vi "Register Listener.vi"(8 "error in (no error)":errorcluster, 10 "Actor's Enqueuer":refnum<class "Message Enqueuer.lvclass">, 11 "Trace Controller in":refnum<class "Trace Controller.lvclass">) -> (0 "error out":errorcluster, 3 "Trace Controller out":refnum<class "Trace Controller.lvclass">)   [LabVIEW 2014, in "Robot Actor Framework.lvlib" / "Trace.lvlib" / "Trace Controller.lvclass"]
uses:
  Trace Controller.lvclass
  <vilib>/ActorFramework/Message Enqueuer/Message Enqueuer.lvclass
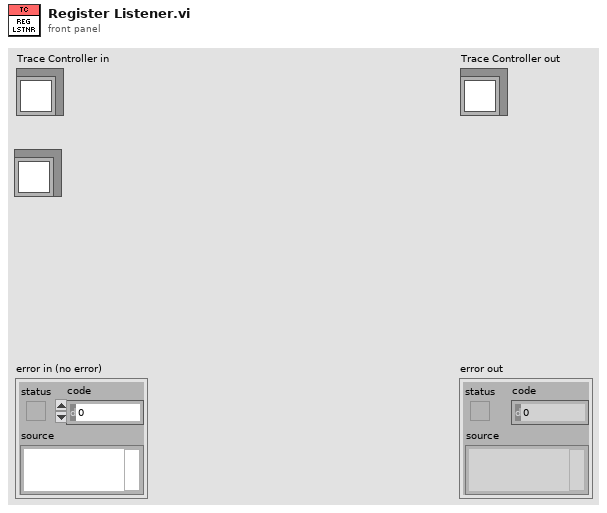
[diagram p1: front panel]
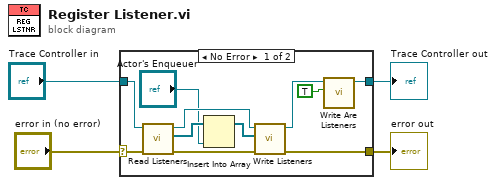
[diagram p0: block diagram]
diagram:
  n1 = case shown="No Error" "error in (no error)" {
    selector: "error in (no error)" -> [w11 w17]
    tunnel: [w9 w17] -> w3
    tunnel: [w7 w16] -> w1
    tunnel: "Trace Controller in" -> [w12 w16]
    frame No Error {
      n2 = call-dynamic "Read Listeners.vi"("error in (no error)"=w11, "Trace Controller in"=w12) -> ("error out"=w10:errorcluster, "Listeners"=w14:refnum<class "Message Enqueuer.lvclass">[], "Trace Controller out"=w15:refnum<class "Trace Controller.lvclass">)  [unwired: 7 in]
      n3 = Insert Into Array(array=w14, new element="Actor's Enqueuer") -> (w13:refnum<class "Message Enqueuer.lvclass">[])  [unwired: 1 in]
      n4 = call-dynamic "Write Listeners.vi"("error in (no error)"=w10, "Listeners"=w13, "Trace Controller in"=w15) -> ("error out"=w9:errorcluster, "Trace Controller out"=w8:refnum<class "Trace Controller.lvclass">)  [unwired: 7 in]
      n5 = call-dynamic "Write Are Listeners.vi"("Are Listeners?"=TRUE, "Trace Controller in"=w8) -> ("Trace Controller out"=w7:refnum<class "Trace Controller.lvclass">)  [unwired: 8 in, 1 out]
    }
    frame Error {
    }
  }
  "error out" <- w3
  "Trace Controller out" <- w1
